vi "subGenerateListToOrder2.vi"(8 "error in (no error)":errorcluster, 11 "SolutionBuilder in":refnum<class "SolutionBuilder.lvclass">) -> (0 "error out":errorcluster, 1 "Ordering map":T1, 3 "SolutionBuilder out":refnum<class "SolutionBuilder.lvclass">)   [LabVIEW 2019, in "SolutionBuilder.lvlib" / "SolutionBuilder.lvclass"]
uses:
  SolutionBuilder.lvclass
  OrderingMap.ctl
  ProjectItem/ProjectItem.lvclass
  ProjectItem/ProjectItem.lvclass/ProjectItem.ctl
  <vilib>/Utility/miscctls.llb/LVMapReplaceAction.ctl
  be8949a1-daf6-466d-868e-55db06778a0f.vi
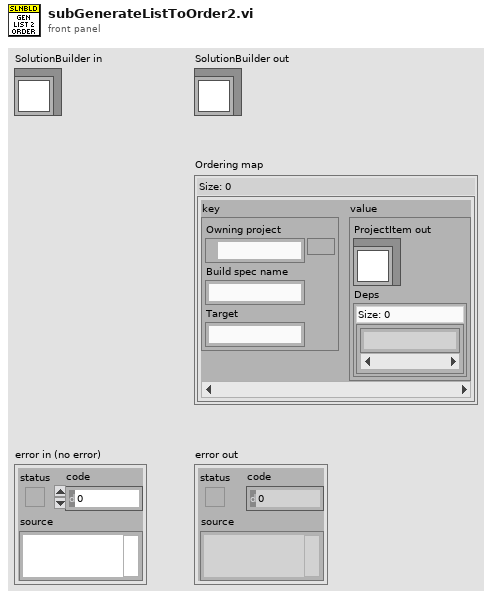
[diagram p1: front panel]
types:
  T1 = typedef "SolutionBuilder.lvlib/SolutionBuilder.lvclass/OrderingMap.ctl" = map{cluster{"Owning project":path, "Build spec name":string, "Target":string}, cluster{"ProjectItem out":refnum<class "ProjectItem.lvclass">, "Deps":set{string}}}
  T2 = typedef "SolutionBuilder.lvlib/SolutionBuilder.lvclass/ProjectItemMap.ctl" = map{path, refnum<class "ProjectItem.lvclass">[]}
  T3 = typedef "LVMapReplaceAction.ctl" = enum32{"Modify Entry only if found", "Add or Modify Entry", "Delete Entry"}
  T4 = cluster{"Owning project":path, "Build spec name":string, "Target":string}
  T5 = cluster{"ProjectItem out":refnum<class "ProjectItem.lvclass">, "Deps":set{string}}
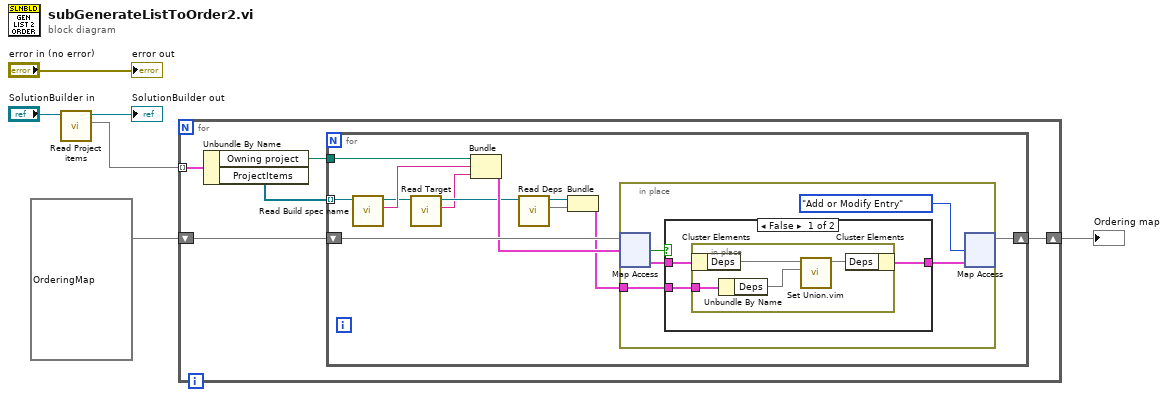
[diagram p0: block diagram]
diagram:
  n1 = call-dynamic "Read Project items.vi"("SolutionBuilder in"="SolutionBuilder in") -> ("Project items"=w1:T2, "SolutionBuilder out"=→"SolutionBuilder out":refnum<class "SolutionBuilder.lvclass">)  [unwired: 9 in]
  n2 = for {
    tunnel: w1 -> [w11] mode=indexing
    shift-right: [w7] -> w4
    shift-left: T1 {} ("Ordering map") -> [w8]
    n3 = Unbundle By Name(w11) -> ("Owning project"=w10:path, "ProjectItems"=w9:refnum<class "ProjectItem.lvclass">[])
    n4 = for {
      tunnel: w9 -> [w23] mode=indexing
      tunnel: w10 -> [w19]
      shift-right: [w15] -> w7
      shift-left: w8 -> [w18]
      n5 = call-dynamic "Read Build spec name.vi"("ProjectItem in"=w23) -> ("Build spec name"=w22:string, "ProjectItem out"=w14:refnum<class "ProjectItem.lvclass">)  [unwired: 9 in]
      n6 = call "Read Target.vi"("ProjectItem in"=w14) -> ("Target"=w12:string, "ProjectItem out"=w13:refnum<class "ProjectItem.lvclass">)  [unwired: 9 in]
      n7 = Bundle("Owning project"=w19, "Build spec name"=w22, "Target"=w12) -> (w17:T4)  [unwired: 1 in]
      n8 = call-dynamic "Read Deps.vi"("ProjectItem in"=w13) -> ("Deps"=w20:set{string}, "ProjectItem out"=w21:refnum<class "ProjectItem.lvclass">)  [unwired: 9 in]
      n9 = Bundle("ProjectItem out"=w21, "Deps"=w20) -> (w16:T5)  [unwired: 1 in]
      n10 = in-place {
        in-place-border: w16 -> [w27]
        n11 = in-place-map #1(w18, w17) -> (w24:T5, w28:bool)  [unwired: 1 in]
        n12 = case shown="False" w28 {
          tunnel: w27 -> [w30 w36]
          tunnel: [w29 w36] -> w26
          tunnel: w24 -> [w31 _]
          frame False {
            n13 = in-place {
              in-place-border: w30 -> [w35]
              n14 = in-place-cluster #2(w31) -> ("Deps"=w34:set{string})
              n15 = Unbundle By Name(w35) -> ("Deps"=w33:set{string})
              n16 = call "Set Union.vim"("set 2"=w33, "set 1"=w34) -> ("union"=w32:set{string})  [unwired: 9 in]
              n17 = in-place-cluster #2("Deps"=w32) -> (w29:T5)
            }
          }
          frame True {
          }
        }
        n18 = in-place-map #1(w26, LVMapReplaceAction."Add or Modify Entry" ("action")) -> (w15:T1)  [unwired: 2 out]
      }
    }
  }
  "Ordering map" <- w4
  "error out" <- "error in (no error)"
